vi "Valid Guesses--constant.vi"() -> (2 "Valid Guesses (array)":string[](array[string]), 3 "Valid Guesses (set)":set{string}(c389))   [LabVIEW 2020, in "Wordle Engine.lvlib"]
doc: "All valid guesses for the Wordle word. The target word was selected from an undisclosed subset of the words in this list.\n\nNote that this VI returns the list as both an array of strings, and a set of strings."
uses:
  Wordle Engine.lvlib
  d1d68809-3a0a-41f9-9956-b3f279d726ed.vi
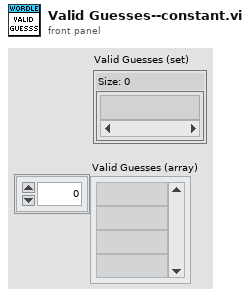
[diagram p1: front panel]
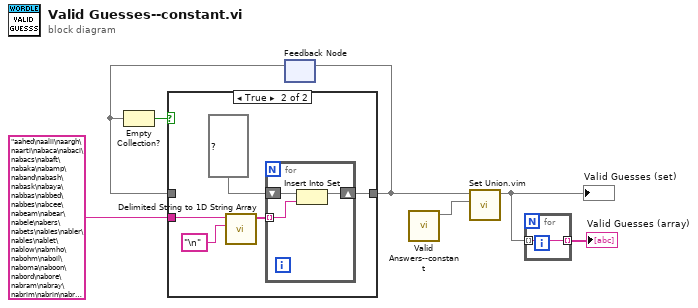
[diagram p0: block diagram]
diagram:
  n1 = feedback #1() -> (w5:set{string})  [unwired: 1 in]
  n2 = Empty Collection?(1:w5) -> (0:w7:bool)
  n3 = case shown="True" w7 {
    tunnel: "aahed\naalii\naargh\naarti\nabaca\nabaci\nabacs\nabaft\nabaka\nabamp\naband\nabash\nabask\nabaya\nabbas\nabbed\nabbes\nabcee\nabeam\nabear\nabele\nabers\nabets\nabies\nabler\nables\nablet\nablow\nabmho\nabohm\naboil\naboma\naboon\nabord\nabore\nabram\nabray\nabrim\nabrin\nabris\nabsey\nabsit\nabuna\nabune\nabuts\nabuzz\nabyes\nabysm\nacais\nacari\naccas\naccoy\nacerb\nacers\naceta\nachar\nached\naches\nachoo\nacids\nacidy\nacing\nacini\nackee\nacker\nacmes\nacmic\nacned\nacnes\nacock\nacold\nacred\nacres\nacros\nacted\nactin\nacton\nacyls\nadaws\nadays\nadbot\naddax\nadded\nadder\naddio\naddle\nadeem\nadhan\nadieu\nadios\nadits\nadman\nadmen\nadmix\nadobo\nadown\nadoze\nadrad\nadred\nadsum\n..." -> [_ w13]
    tunnel: [w8 w10] -> w4
    tunnel: w5 -> [w8 _]
    frame False {
    }
    frame True {
      n4 = call <vilib>:"Delimited String to 1D String Array.vi"("delimiter"="\n", "delimited string"=w13) -> ("string array"=w12:string[])  [unwired: 9 in]
      n5 = for {
        tunnel: w12 -> [w14] mode=indexing
        shift-right: [w16] -> w10
        shift-left: set{string} {} ("Valid Guesses") -> [w15]
        n6 = Insert Into Set(10:w14, 11:w15) -> (3:w16:set{string})  [unwired: 1 out]
      }
    }
  }
  n7 = feedback-in #1(w4) -> ()
  n8 = call "Valid Answers--constant.vi"() -> ("Valid Answers"=w3:set{string})  [unwired: 11 in]
  n9 = call "Set Union.vim"("set 2"=w3, "set 1"=w4) -> ("union"=w2:set{string})  [unwired: 9 in]
  "Valid Guesses (set)" <- w2
  n10 = for {
    tunnel: [w17] -> w1 mode=indexing
    tunnel: w2 -> [w17] mode=indexing
  }
  "Valid Guesses (array)" <- w1
